vi "Write Config info.vi"(10 "Config info":T1={"RBW"=0.0, "VBW "=0.0, "Number of Averages"=0.0, "Average On"=FALSE, "Frequency (MHz)"="900", "Offset Frequency (MHz)"="45", "Power (dBm)"="20:30/2", "Delta Power (dB)"="20:30/2", "Uneven IMD"=FALSE, "Loop order"=enum."Device -> Power -> Frequency -> Offset", "Stop level"=999.0, "IMD2"=FALSE, "IMD3"=FALSE}, 11 "IMD in":refnum<class "IMD.lvclass">) -> (3 "IMD out":refnum<class "IMD.lvclass">)   [LabVIEW 2020, in "IMD.lvclass"]
uses:
  IMD.lvclass
  Controls/Config info.ctl
  Controls/Loop order.ctl
  IMD.lvclass/IMD.ctl
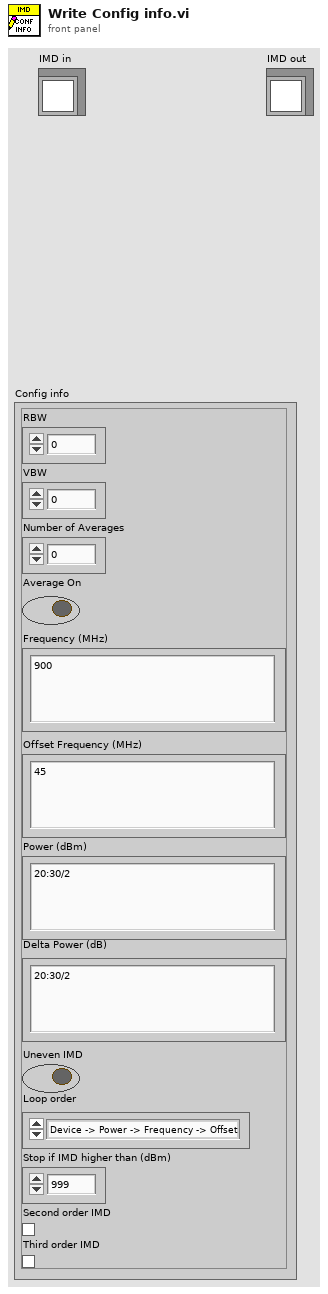
[diagram p1: front panel]
types:
  T1 = typedef "IMD.lvclass/Config info.ctl" = cluster{"RBW":dbl, "VBW ":dbl, "Number of Averages":dbl, "Average On":bool, "Frequency (MHz)":string, "Offset Frequency (MHz)":string, "Power (dBm)":string, "Delta Power (dB)":string, "Uneven IMD":bool, "Loop order":T2, "Stop level":dbl, "IMD2":bool, "IMD3":bool}
  T2 = typedef "IMD.lvclass/Loop order.ctl" = enum16{"Device -> Power -> Frequency -> Offset", "Device -> Frequency -> Power -> Offset"}
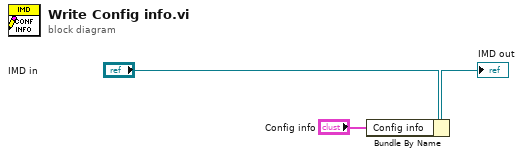
[diagram p0: block diagram]
diagram:
  n1 = Bundle By Name(cluster="IMD in", "Config info"="Config info") -> (→"IMD out":refnum<class "IMD.lvclass">)
